vi "Max and Min (single).vi"(8 "error in (no error)":errorcluster, 11 "XY-data":cluster{"X-array":dbl[], "Y-array":dbl[]} {"Y-array" format="%.2p"; "X-array" format="%.2p"}) -> (0 "error out":errorcluster, 1 "y_min (x,y)":cluster{"x":dbl, "y":dbl}, 2 "y_max (x,y)":cluster{"x":dbl, "y":dbl}, 3 "XY-data out":cluster{"X-array":dbl[], "Y-array":dbl[]} {"Y-array" format="%.2p"; "X-array" format="%.2p"})   [LabVIEW 2019, in "xy_utilities.lvlib"]
doc: "Returns (x,y) coordinates of <b>y_max</b> and <b>y_min</b>.\n\nWire data to the data input to determine the polymorphic instance to use or manually select the instance."
uses:
  xy_utilities.lvlib
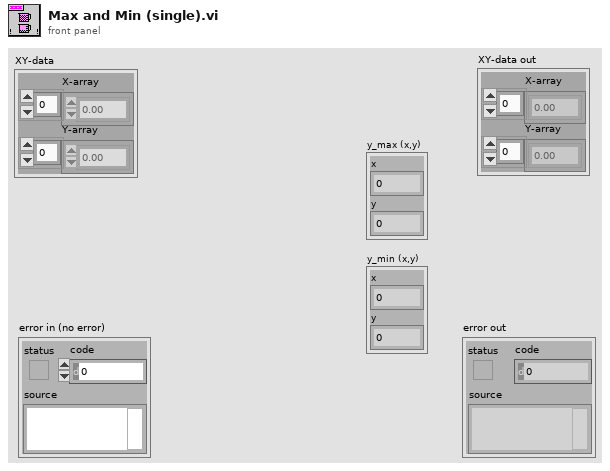
[diagram p1: front panel]
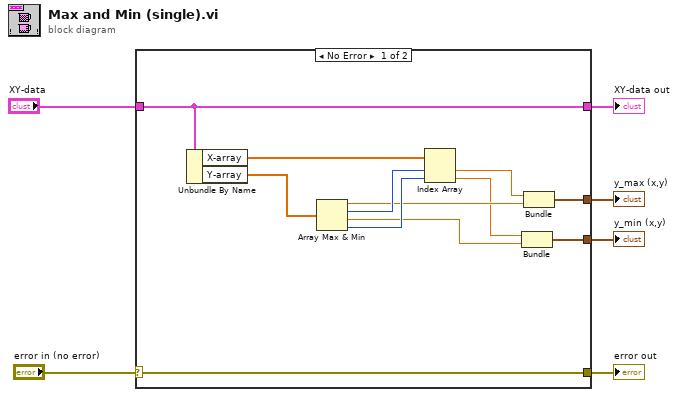
[diagram p0: block diagram]
diagram:
  n1 = case shown="No Error" "error in (no error)" {
    selector: "error in (no error)" -> [w18 w20]
    tunnel: [w18 w20] -> w5
    tunnel: "XY-data" -> [w7 w19]
    tunnel: [w7 w19] -> w3
    tunnel: [w11 _] -> w2
    tunnel: [w8 _] -> w1
    frame No Error {
      n2 = Unbundle By Name(w7) -> ("X-array"=w16:dbl[], "Y-array"=w15:dbl[])
      n3 = Array Max & Min(array=w15) -> (max value=w12:dbl, max index (indices)=w17:i32, min value=w9:dbl, min index (indices)=w14:i32)
      n4 = Index Array(array=w16, index #1=w17, index #2=w14) -> (element #1=w13:dbl, element #2=w10:dbl)
      n5 = Bundle("x"=w10, w9) -> (w8:cluster{"x":dbl, dbl})  [unwired: 1 in]
      n6 = Bundle("x"=w13, w12) -> (w11:cluster{"x":dbl, dbl})  [unwired: 1 in]
    }
    frame Error {
    }
  }
  "error out" <- w5
  "XY-data out" <- w3
  "y_max (x,y)" <- w2
  "y_min (x,y)" <- w1
